vi "Trigger.vi"(8 "error in (no error)":errorcluster, 11 "VISA resource name":refnum<visa-resource-name>) -> (0 "error out":errorcluster, 3 "VISA resource name out":refnum<visa-resource-name>)   [LabVIEW 2021, in "Sorensen M9A Series.lvlib"]
doc: "This VI first checks to see if the Sorensen power supply is in hold mode. If it is, then the trigger command is sent, so that the most recent current and voltage settings are applied. If the power supply is not in hold mode, then this VI does nothing."
uses:
  Sorensen M9A Series.lvlib
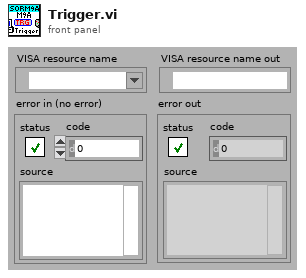
[diagram p1: front panel]
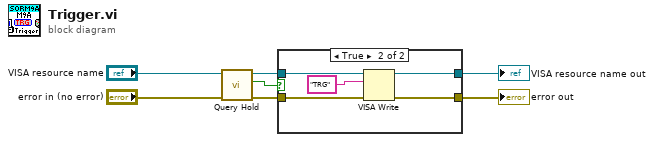
[diagram p0: block diagram]
diagram:
  n1 = call "Query Hold.vi"("error in (no error)"="error in (no error)", "VISA resource name"="VISA resource name") -> ("error out"=w1:errorcluster, "Hold?"=w3:bool, "VISA resource name out"=w2:refnum<visa-resource-name>)  [unwired: 7 in]
  n2 = case shown="True" w3 {
    tunnel: w2 -> [w9 w13]
    tunnel: w1 -> [w8 w12]
    tunnel: [w9 w11] -> w7
    tunnel: [w8 w10] -> w6
    frame False {
    }
    frame True {
      n3 = VISA Write(VISA resource name=w13, write buffer="TRG" ("data"), error in (no error)=w12) -> (VISA resource name out=w11:refnum<visa-resource-name>, error out=w10:errorcluster)  [unwired: 1 out]
    }
  }
  "error out" <- w6
  "VISA resource name out" <- w7
